vi "Features_SpecPage.vi"(10 "Spec Page Interface":T2, 11 "MetaDataObj in":refnum<class "MetaDataObj.lvclass">) -> (3 "MetaDataObj out":refnum<class "MetaDataObj.lvclass">)   [LabVIEW 2013, in "TagBusConfigurablePluginDecideFeatures.lvclass"]
uses:
  TagBusConfigurablePluginDecideFeatures.lvclass
  <resource>/dialog/NewProjectWizard/Spec Page Interface.ctl
  <resource>/dialog/NewProjectWizard/MetaDataObj/MetaDataObj.lvclass
  <resource>/dialog/NewProjectWizard/MetaDataObj/MetaDataObj.lvclass/MetaDataObj.ctl
  TagBusConfigurablePluginDecideFeatures.lvclass/TagBusConfigurablePluginDecideFeatures.ctl
  <vilib>/NI/Tag Bus Module Framework/root configuration/Target Types.ctl
  <vilib>/NI/Tag Bus/tag/Data Type.ctl
  <resource>/dialog/NewProjectWizard/MetaDataObj/Accessors/Write Project Name.vi
  <resource>/dialog/NewProjectWizard/MetaDataObj/Accessors/Write Project Root.vi
  Write component name.vi
  Write supported targets.vi
  Write supported data types.vi
  Write instances allowed.vi
  <resource>/dialog/NewProjectWizard/MetaDataObj/Accessors/Write File Prefix.vi
  <vilib>/NI/Tag Bus/tag/count types.vi
  <vilib>/NI/Tag Bus/tag/index to type.vi
  <vilib>/NI/Tag Bus Module Framework/root configuration/TBM configuration.lvclass
  <vilib>/NI/Tag Bus/tag/tag descriptor.lvclass
panel:
  in  "Tab Control":T1(tab)
  in  "Instances Allowed":i32=-1
  in  "Supported Targets":i32[](listbox)
  in  "Available Targets":i32[](listbox)
  in  "+target":bool
  in  "-target":bool
  in  "-type":bool
  in  "+type":bool
  in  "Available Data Types":i32[](listbox)
  in  "Supported Data Types":i32[](listbox)
  in  "Component Name":string
  in  "Project Root":path
  # "Execution Behaviors:"
  # "Number of classes allowed in a system. Default is infinite, -1. Examples: {Scaling: -1};{Scan Engine: 1}"
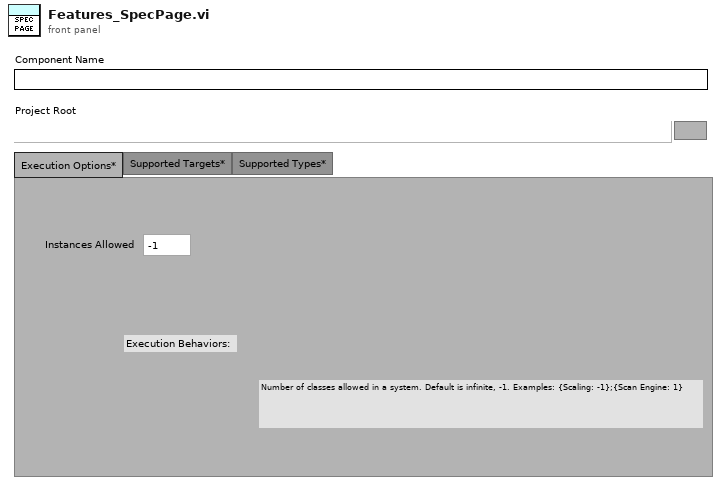
[diagram p1: front panel]
types:
  T1 = enum32{"Execution Options*", "Supported Targets*", "Supported Types*"}
  T2 = typedef "Spec Page Interface.ctl" = cluster{"\"Tab Forward To\" Refnum":refnum<vi>, "\"Tab Backward To\" Refnum":refnum<vi>, "Errors":refnum<user-event>, "Quit":refnum<user-event>}
  T3 = typedef "TBM configuration.lvclass/Target Types.ctl" = enum16{"Windows", "Mac", "Linux", "Linux RT ARM", "VxWorks", "Pharlap", "Other", "Linux RT x64"}
  T4 = typedef "tag bus.lvlib/tag descriptor.lvclass/Data Type.ctl" = enum16{"Double", "Single", "I64", "I32", "I16", "I8", "U64", "U32", "U16", "U8", "Boolean", "String", "Array of Double", "Array of Single", "Array of I64", "Array of I32", "Array of I16", "Array of I8", "Array of U64", "Array of U32", "Array of U16", "Array of U8", "Array of Boolean", "Array of String"}
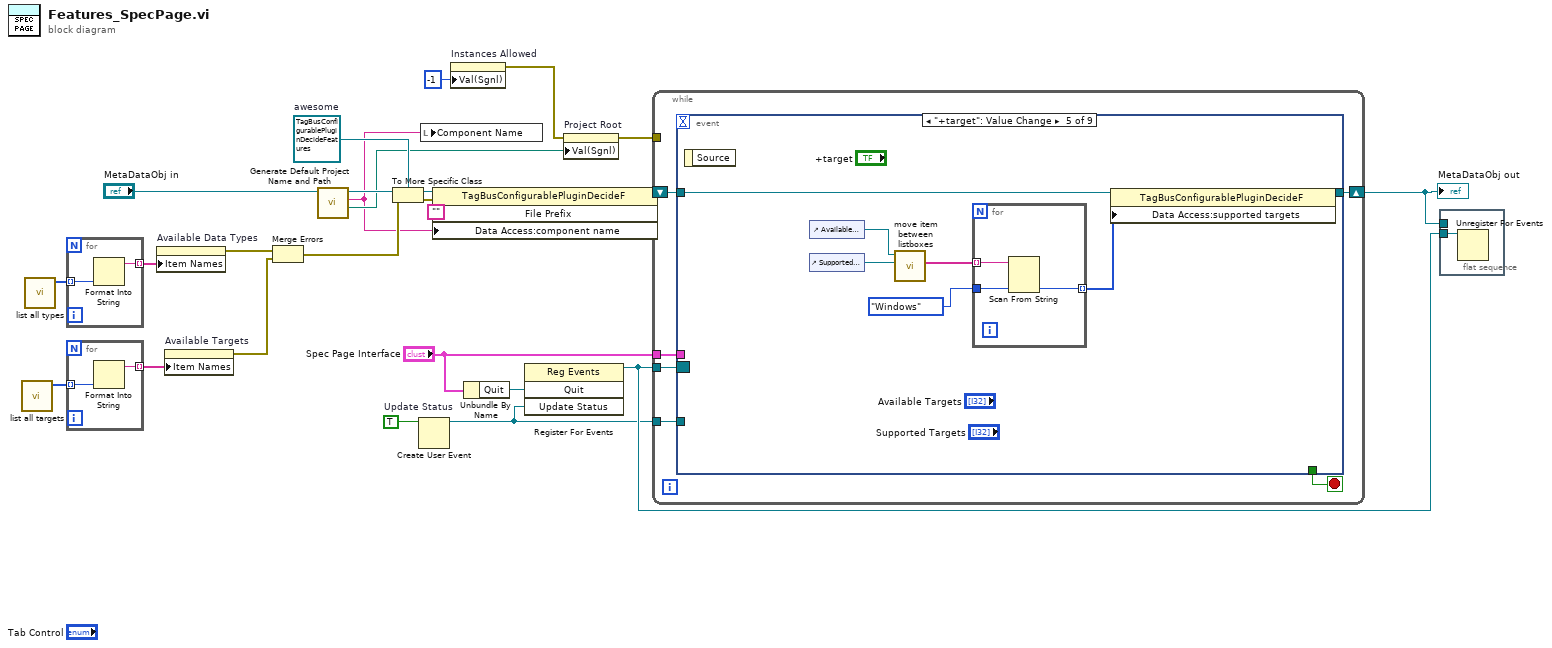
[diagram p0: block diagram]
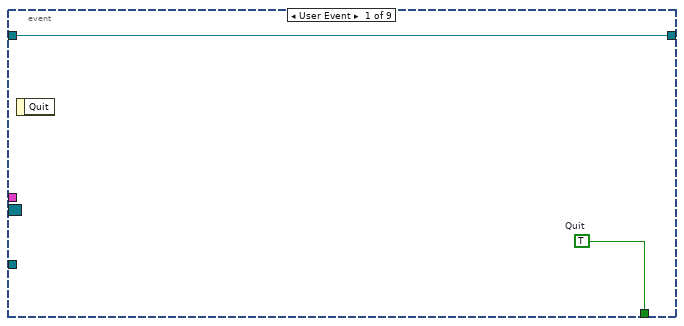
[diagram p2: hidden frame]
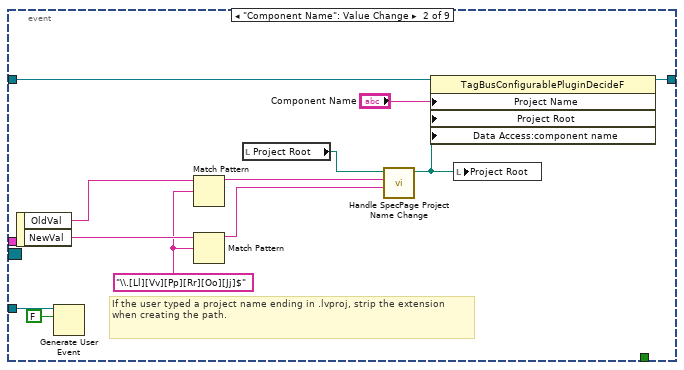
[diagram p3: hidden frame]
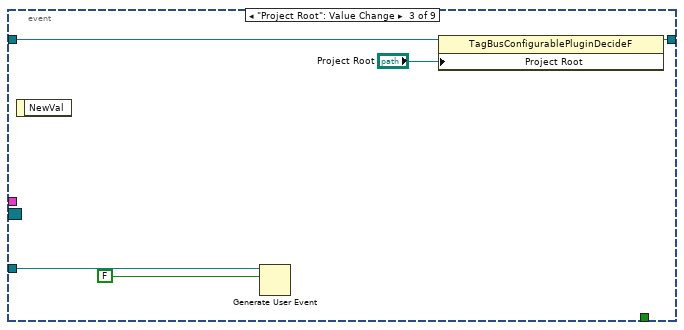
[diagram p4: hidden frame]
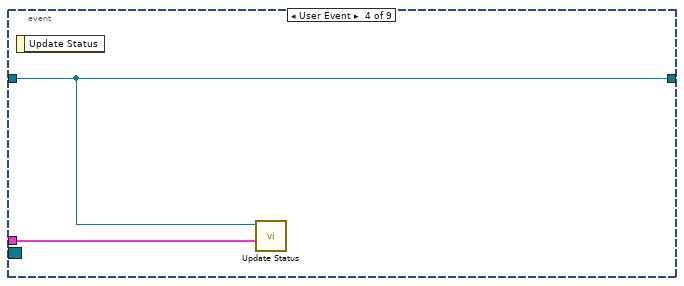
[diagram p5: hidden frame]
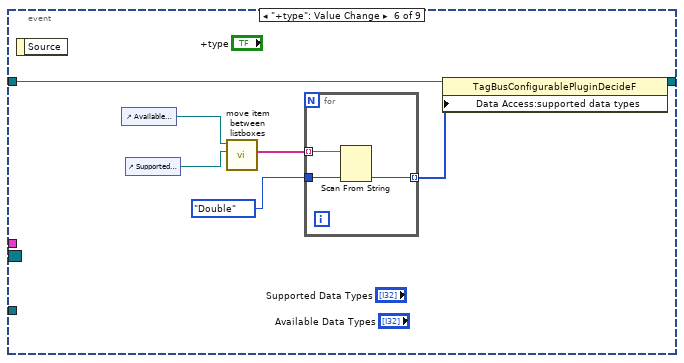
[diagram p6: hidden frame]
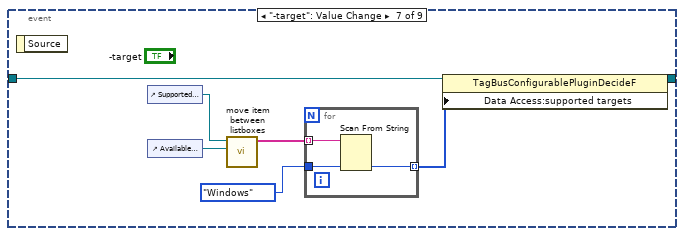
[diagram p7: hidden frame]
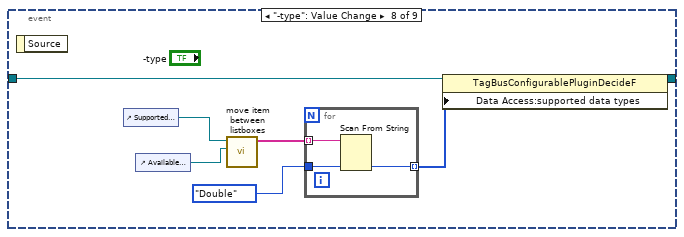
[diagram p8: hidden frame]
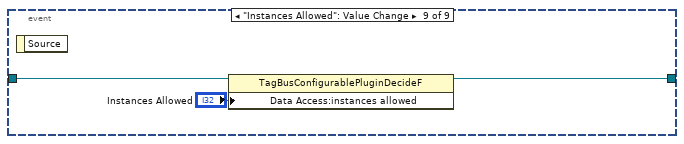
[diagram p9: hidden frame]
diagram:
  w19 = TRUE  # Update Status
  w20 = refnum<class "TagBusConfigurablePluginDecideFeatures.lvclass"> refnum  # awesome
  n1 = call <vilib>:"list all targets.vi"() -> ("all targets"=w9:T3[])  [unwired: 11 in]
  n2 = call <vilib>:"list all types.vi"() -> ("all types"=w11:T4[])  [unwired: 11 in]
  n3 = for {
    tunnel: w11 -> [w27] mode=indexing
    tunnel: [w26] -> w10 mode=indexing
    n4 = Format Into String(w27) -> (resulting string=w26:string)  [unwired: 3 in, 1 out]
  }
  n5 = for {
    tunnel: w9 -> [w29] mode=indexing
    tunnel: [w28] -> w8 mode=indexing
    n6 = Format Into String(w29) -> (resulting string=w28:string)  [unwired: 3 in, 1 out]
  }
  n7 = property on="Available Data Types" class="LstBox (strict)"("Item Names"=w10) -> (error out=w7:errorcluster)  [unwired: 2 in, 1 out]
  n8 = property on="Available Targets" class="LstBox (strict)"("Item Names"=w8) -> (error out=w6:errorcluster)  [unwired: 2 in, 1 out]
  n9 = Merge Errors(w7, w6) -> (w5:errorcluster)
  n10 = call <resource>:"Generate Default Project Name and Path.vi"("DNL_MetaDataObj in"="MetaDataObj in") -> ("Project Root"=w12:path, "Project Name"=w3:string, "DNL_MetaDataObj out"=w13:refnum<class "MetaDataObj.lvclass">)  [unwired: 8 in]
  n11 = To More Specific Class(target class=w20, reference=w13, error in=w5) -> (specific class reference=w22:refnum<class "TagBusConfigurablePluginDecideFeatures.lvclass">, error out=w21:errorcluster)
  n12 = Create User Event(user event datatype=w19) -> (user event=w16:refnum<user-event>)  [unwired: 1 in, 1 out]
  n13 = local write "Component Name"(w3) -> ()
  n14 = property class="TagBusConfigurablePluginDecideF"(reference=w22, error in=w21, "File Prefix"="", "Data Access:component name"=w3) -> (reference out=w18:refnum<class "TagBusConfigurablePluginDecideFeatures.lvclass">)  [unwired: 1 out]
  n15 = property on="Instances Allowed" class="DigNum (strict)"("Val(Sgnl)"=-1 ("Value (Signaling)")) -> (error out=w2:errorcluster)  [unwired: 2 in, 1 out]
  n16 = Unbundle By Name("Spec Page Interface") -> ("Quit"=w25:refnum<user-event>)
  n17 = register-events(w25, w16) -> (reference out=w24:refnum<event-registration>)  [unwired: 2 in, 1 out]
  n18 = property on="Project Root" class="Path"(error in=w2, "Val(Sgnl)"=w12) -> (error out=w17:errorcluster)  [unwired: 1 in, 1 out]
  n19 = while {
    tunnel: "Spec Page Interface" -> [w34]
    shift-right: [w32] -> w4
    shift-left: w18 -> [w31]
    tunnel: w24 -> [w33]
    tunnel: w17 -> [_]
    tunnel: w16 -> [w30]
    stop <- w35 stop-if-true
    n20 = event shown="[4] \"+target\": Value Change" {
      selector: w33 -> [_ _ _ _ _ _ _ _ _]
      dyn-events: _ -> [_ _ _ _ _ _ _ _ _]
      timeout: _ -> [_ _ _ _ _ _ _ _ _]
      tunnel: w34 -> [_ _ _ w55 _ _ _ _ _]
      tunnel: [w37 _ _ _ _ _ _ _ _] -> w35
      tunnel: [w36 w49 w53 w56 w62 w72 w82 w92 w98] -> w32
      tunnel: w31 -> [w36 w46 w54 w56 w63 w73 w83 w93 w99]
      tunnel: w30 -> [_ w48 w52 _ _ _ _ _ _]
      event User Event {
        w37 = TRUE  # Quit
        n21 = event-data() -> ()  [unwired: 1 in, 1 out]
      }
      event "Component Name": Value Change {
        w41 = "\\.[Ll][Vv][Pp][Rr][Oo][Jj]$" ("regular expression")
        # "If the user typed a project name ending in .lvproj, strip the extension when creating the path."
        n22 = event-data() -> ("OldVal"=w43:string, "NewVal"=w42:string)  [unwired: 1 in]
        n23 = Generate User Event(user event=w48, event data cluster=FALSE ("Update Status")) -> ()  [unwired: 2 in, 2 out]
        n24 = Match Pattern(string=w43, regular expression=w41) -> (before substring=w40:string)  [unwired: 1 in, 3 out]
        n25 = Match Pattern(string=w42, regular expression=w41) -> (before substring=w39:string)  [unwired: 1 in, 3 out]
        n26 = local read "Project Root"() -> (w45:path)
        n27 = call <resource>:"Handle SpecPage Project Name Change.vi"("Project Name New Value"=w39, "Project Name Old Value"=w40, "Project Root in"=w45) -> ("Project Root out"=w44:path)  [unwired: 8 in]
        n28 = property class="TagBusConfigurablePluginDecideF"(reference=w46, "Project Name"="Component Name", "Project Root"=w44, "Data Access:component name"="Component Name") -> (reference out=w49:refnum<class "TagBusConfigurablePluginDecideFeatures.lvclass">)  [unwired: 1 in, 1 out]
        n29 = local write "Project Root"(w44) -> ()
      }
      event "Project Root": Value Change {
        n30 = event-data() -> ()  [unwired: 1 in, 1 out]
        n31 = Generate User Event(user event=w52, event data cluster=FALSE ("Update Status")) -> ()  [unwired: 2 in, 2 out]
        n32 = property class="TagBusConfigurablePluginDecideF"(reference=w54, "Project Root"="Project Root") -> (reference out=w53:refnum<class "TagBusConfigurablePluginDecideFeatures.lvclass">)  [unwired: 1 in, 1 out]
      }
      event User Event {
        n33 = event-data() -> ()  [unwired: 1 in, 1 out]
        n34 = call "Update Status.vi"("Spec Page Interface"=w55, "TwoTasksMetaDataObj in"=w56) -> ()  [unwired: 10 in]
      }
      event "+target": Value Change {
        n35 = event-data() -> ()  [unwired: 1 in, 1 out]
        n36 = control-ref of="Available Targets"() -> (w61:refnum<vi>)
        n37 = control-ref of="Supported Targets"() -> (w60:refnum<vi>)
        n38 = call "move item between listboxes.vi"("target"=w60, "source"=w61) -> ("new target"=w59:string[])  [unwired: 7 in, 2 out]
        n39 = for {
          tunnel: w59 -> [w66] mode=indexing
          tunnel: Target_Types."Windows" ("Target Types") -> [w65]
          tunnel: [w64] -> w57 mode=indexing
          n40 = Scan From String(input string=w66, default 1=w65) -> (output 1=w64:T3)  [unwired: 3 in, 3 out]
        }
        n41 = property class="TagBusConfigurablePluginDecideF"(reference=w63, "Data Access:supported targets"=w57) -> (reference out=w62:refnum<class "TagBusConfigurablePluginDecideFeatures.lvclass">)  [unwired: 1 in, 1 out]
      }
      event "+type": Value Change {
        n42 = event-data() -> ()  [unwired: 1 in, 1 out]
        n43 = control-ref of="Available Data Types"() -> (w67:refnum<vi>)
        n44 = control-ref of="Supported Data Types"() -> (w69:refnum<vi>)
        n45 = call "move item between listboxes.vi"("target"=w69, "source"=w67) -> ("new target"=w71:string[])  [unwired: 7 in, 2 out]
        n46 = for {
          tunnel: w71 -> [w76] mode=indexing
          tunnel: Data_Type."Double" ("Data Type") -> [w75]
          tunnel: [w74] -> w70 mode=indexing
          n47 = Scan From String(input string=w76, default 1=w75) -> (output 1=w74:T4)  [unwired: 3 in, 3 out]
        }
        n48 = property class="TagBusConfigurablePluginDecideF"(reference=w73, "Data Access:supported data types"=w70) -> (reference out=w72:refnum<class "TagBusConfigurablePluginDecideFeatures.lvclass">)  [unwired: 1 in, 1 out]
      }
      event "-target": Value Change {
        n49 = event-data() -> ()  [unwired: 1 in, 1 out]
        n50 = control-ref of="Supported Targets"() -> (w77:refnum<vi>)
        n51 = control-ref of="Available Targets"() -> (w79:refnum<vi>)
        n52 = call "move item between listboxes.vi"("target"=w79, "source"=w77) -> ("new source"=w78:string[])  [unwired: 7 in, 2 out]
        n53 = for {
          tunnel: w78 -> [w86] mode=indexing
          tunnel: Target_Types."Windows" ("Target Types") -> [w85]
          tunnel: [w84] -> w80 mode=indexing
          n54 = Scan From String(input string=w86, default 1=w85) -> (output 1=w84:T3)  [unwired: 3 in, 3 out]
        }
        n55 = property class="TagBusConfigurablePluginDecideF"(reference=w83, "Data Access:supported targets"=w80) -> (reference out=w82:refnum<class "TagBusConfigurablePluginDecideFeatures.lvclass">)  [unwired: 1 in, 1 out]
      }
      event "-type": Value Change {
        n56 = event-data() -> ()  [unwired: 1 in, 1 out]
        n57 = control-ref of="Supported Data Types"() -> (w87:refnum<vi>)
        n58 = control-ref of="Available Data Types"() -> (w88:refnum<vi>)
        n59 = call "move item between listboxes.vi"("target"=w88, "source"=w87) -> ("new source"=w90:string[])  [unwired: 7 in, 2 out]
        n60 = for {
          tunnel: w90 -> [w96] mode=indexing
          tunnel: Data_Type."Double" ("Data Type") -> [w95]
          tunnel: [w94] -> w91 mode=indexing
          n61 = Scan From String(input string=w96, default 1=w95) -> (output 1=w94:T4)  [unwired: 3 in, 3 out]
        }
        n62 = property class="TagBusConfigurablePluginDecideF"(reference=w93, "Data Access:supported data types"=w91) -> (reference out=w92:refnum<class "TagBusConfigurablePluginDecideFeatures.lvclass">)  [unwired: 1 in, 1 out]
      }
      event "Instances Allowed": Value Change {
        n63 = event-data() -> ()  [unwired: 1 in, 1 out]
        n64 = property class="TagBusConfigurablePluginDecideF"(reference=w99, "Data Access:instances allowed"="Instances Allowed") -> (reference out=w98:refnum<class "TagBusConfigurablePluginDecideFeatures.lvclass">)  [unwired: 1 in, 1 out]
      }
    }
  }
  "MetaDataObj out" <- w4
  n65 = flat-sequence {
    tunnel: w24 -> [w100]
    tunnel: w4 -> [_]
    frame #0 {
      n66 = Unregister For Events(event registration refnum=w100) -> ()  [unwired: 1 in, 1 out]
    }
  }
